vi "ProgramWithConsumerAndProducer.vi"() -> ()   [LabVIEW 2020]
uses:
  #typedef_States.ctl
  <vilib>/picture/picture.llb/imagedata.ctl
  #typedef_Database.ctl
  <vilib>/event_ctls.llb/eventvkey.ctl
  shell32.dll
panel:
  in  "EndOfProgram":bool
  in  "BROWSEINFO 2":T1={"hWndOwner"=0, "pidlRoot"=0, "pszDisplayName"=0, "lpszTitle"=0, "ulFlags"=1, "lpfn"=0, "lParam"=0, "iImage"=0}
  in  "List of images":i32[](listbox)
  in  "Path":string
  out "2D Picture":picture
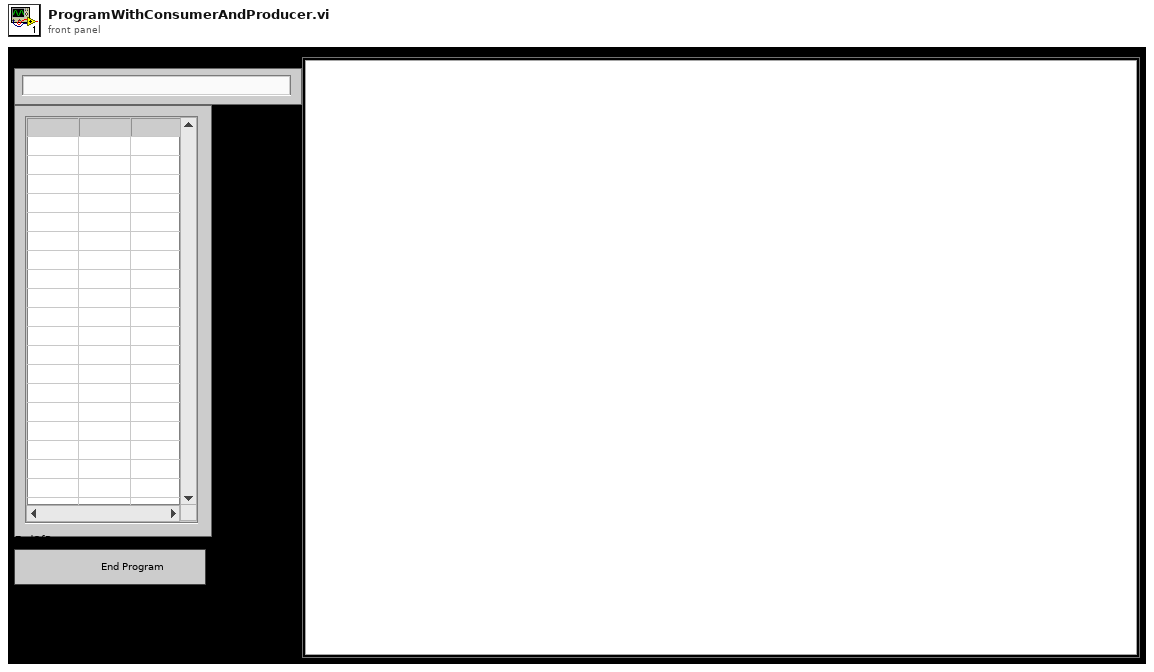
[diagram p1: front panel]
types:
  T1 = cluster{"hWndOwner":i32, "pidlRoot":i32, "pszDisplayName":i32, "lpszTitle":i32, "ulFlags":i32, "lpfn":i32, "lParam":i32, "iImage":i32}
  T2 = typedef "imagedata.ctl" = cluster{"image type":i32, "image depth":i32, "image":u8[], "mask":u8[], "colors":u32[], "Rectangle":cluster{"left":i16, "top":i16, "right":i16, "bottom":i16}}
  T3 = typedef "#typedef_States.ctl" = enum16{"Initialize", "CheckButton", "OpenFromKey", "OpenFromPath", "ImageView", "AreaOfImageResize", "ImageResize", "ChangeImage", "ShowNext", "ShowPrevious", "LoadImagesName", "End"}
  T4 = typedef "#typedef_Database.ctl" = cluster{"Folder Directory":string, "Name of images":string[], "PreviousState":T3, "NumberOfRow":i32, "PanelResizeMeasurement":cluster{"Right":i16, "Left":i16, "Bottom":i16, "Top":i16}, "CurrentImageData":T2, "ImageChangeKey":T5, "IsShiftPressed?":bool}
  T5 = typedef "eventvkey.ctl" = enum16{"ASCII", "Enter", "Return", "Shift", "Ctrl", "Alt", "Cmd", "Opt", "Caps", "NumLock", "Clear", "Break", "Up", "Down", "Left", "Right", "Insert", "Delete", "Home", "End", "PageUp", "PageDown", "Escape", "Help", "Pause", "ScrollLock", "F1", "F2", "F3", "F4", "F5", "F6", "F7", "F8", "F9", "F10", "F11", "F12", "F13", "F14", "F15", "F16", "F17", "F18", "F19", "F20", "F21", "F22", "F23", "F24", "Play", "VolumeUp", "VolumeDown", "Mute", "Two Byte Char"}
  T6 = typedef "LVRectTypeDef.ctl" = cluster{"Left":i16, "Top":i16, "Right":i16, "Bottom":i16}
  T7 = cluster{"Shift":bool, "Ctrl":bool, "Alt":bool, "Cmd":bool, "Opt":bool}
  T8 = typedef "LVBoundsTypeDef.ctl" = cluster{"Width":u32, "Height":u32}
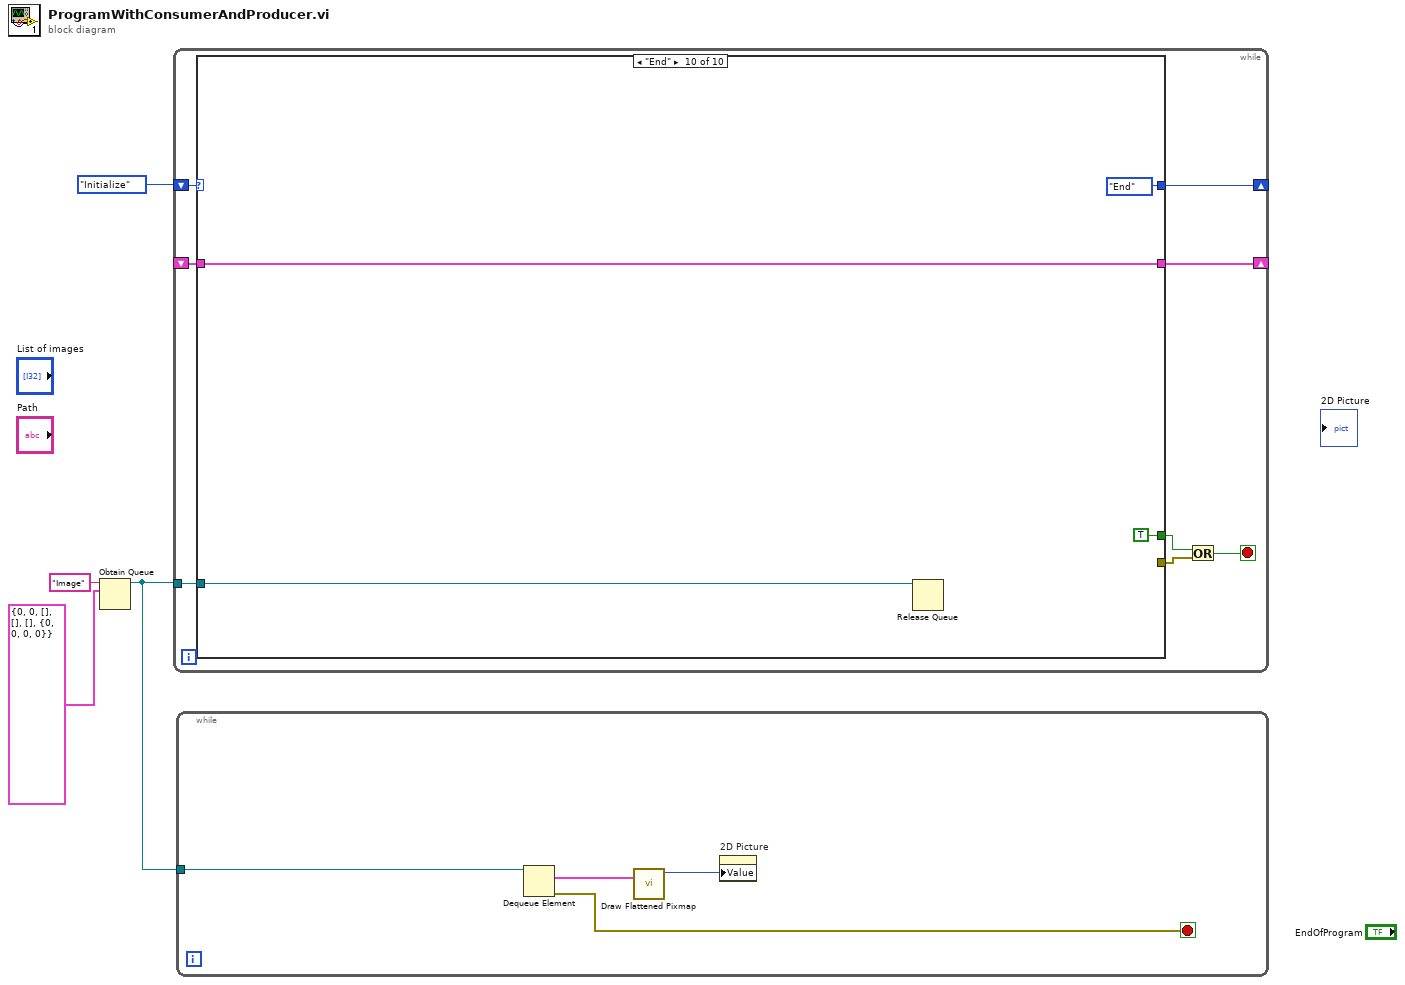
[diagram p0: block diagram]
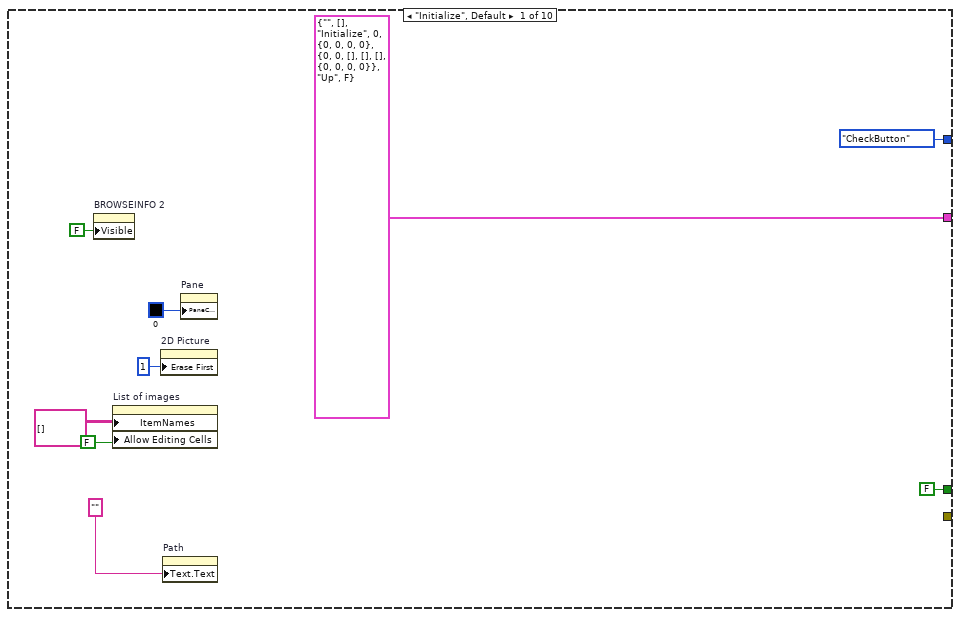
[diagram p2: hidden frame]
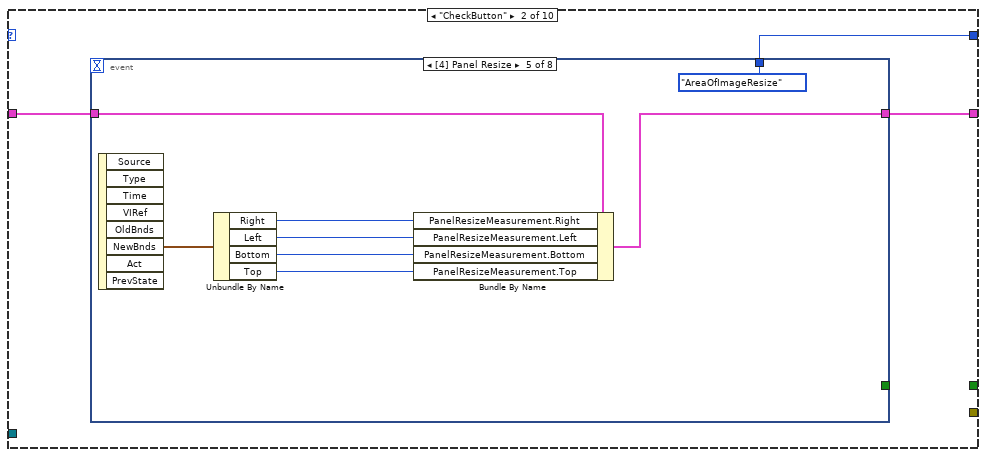
[diagram p3: hidden frame]
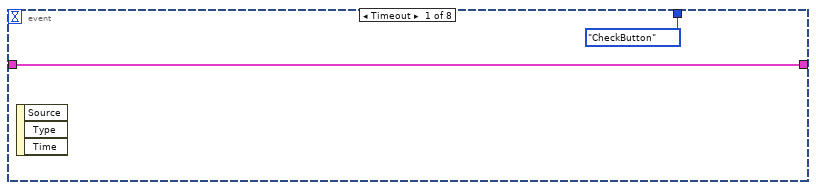
[diagram p4: hidden frame]
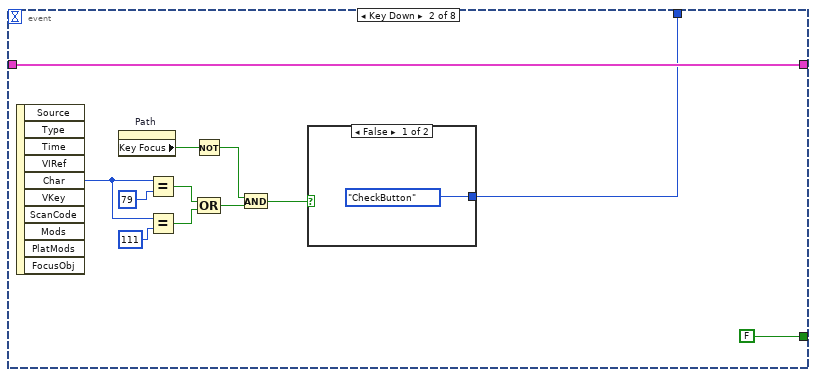
[diagram p5: hidden frame]
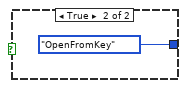
[diagram p6: hidden frame]
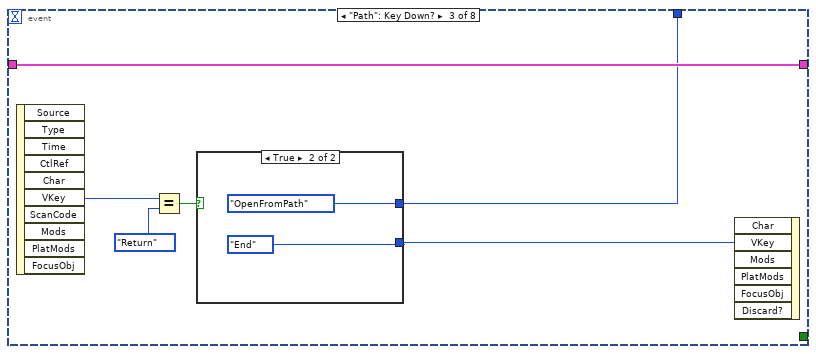
[diagram p7: hidden frame]
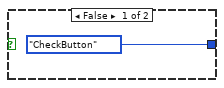
[diagram p8: hidden frame]
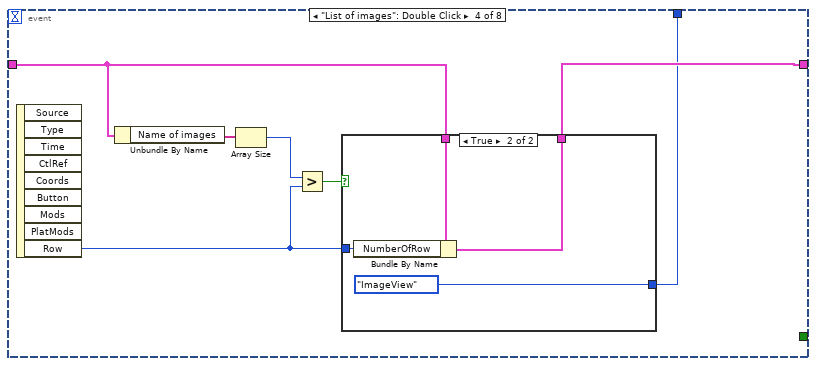
[diagram p9: hidden frame]
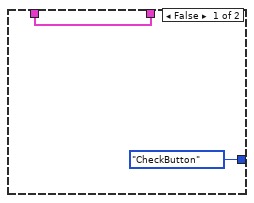
[diagram p10: hidden frame]
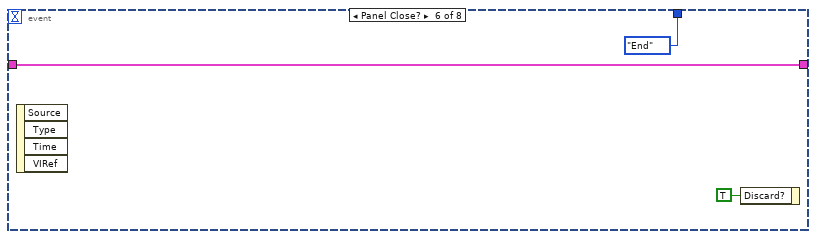
[diagram p11: hidden frame]
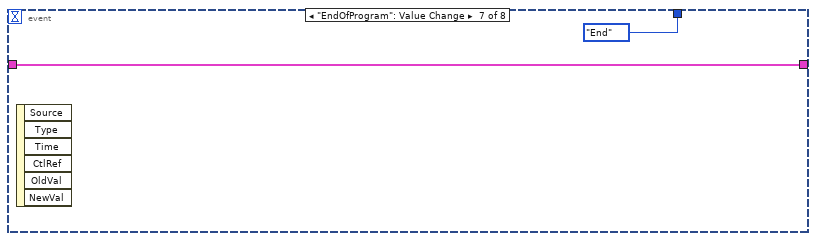
[diagram p12: hidden frame]
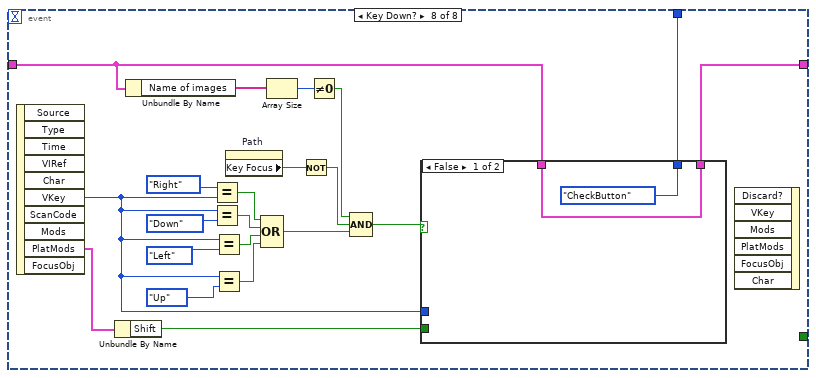
[diagram p13: hidden frame]
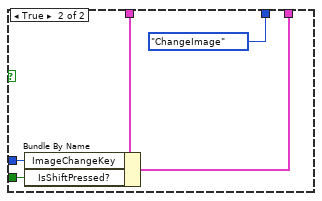
[diagram p14: hidden frame]
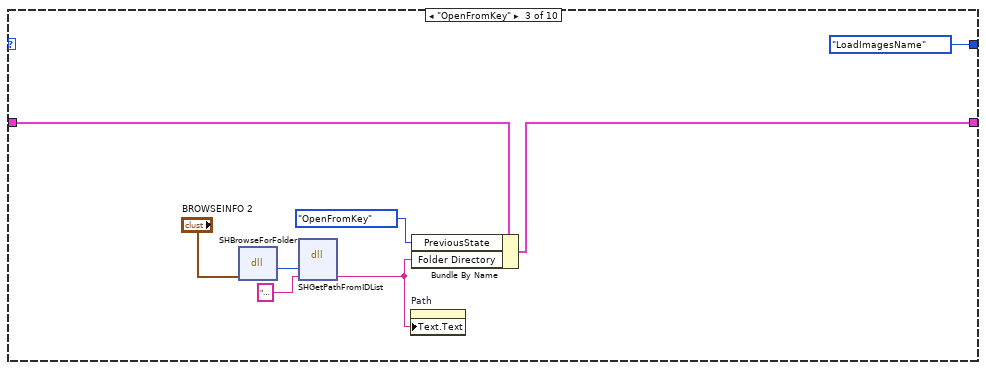
[diagram p15: hidden frame]
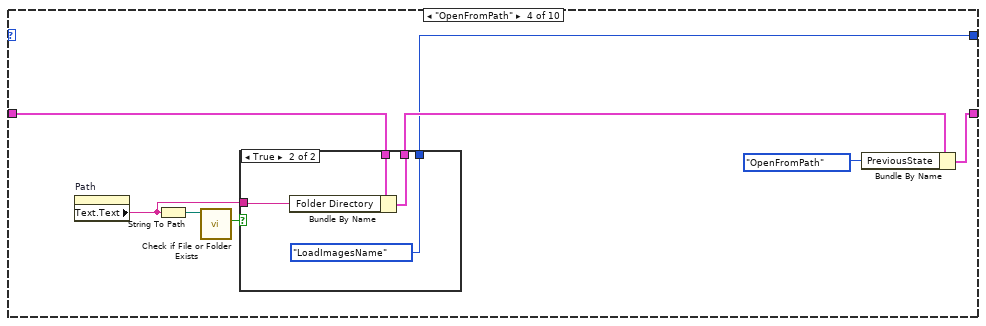
[diagram p16: hidden frame]
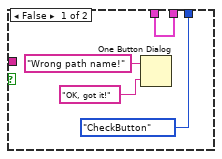
[diagram p17: hidden frame]
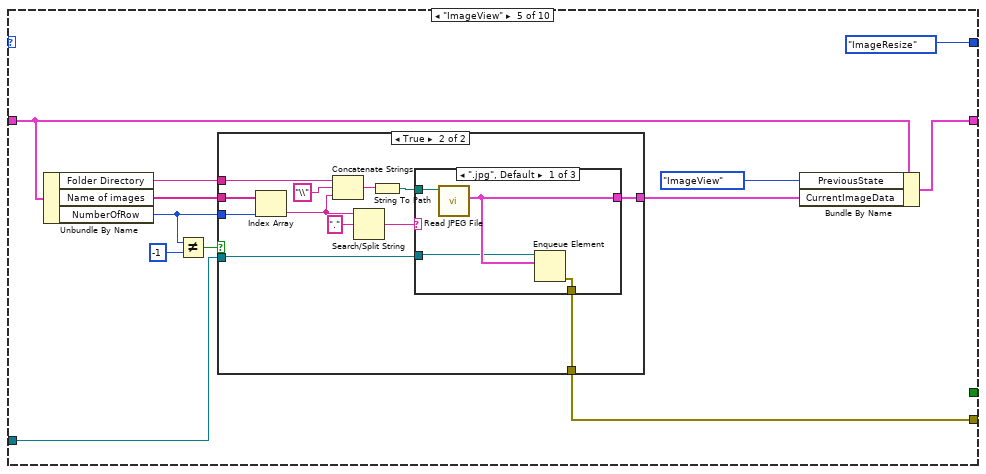
[diagram p18: hidden frame]
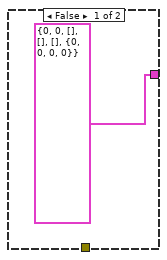
[diagram p19: hidden frame]
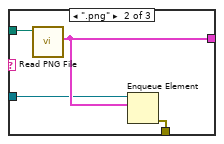
[diagram p20: hidden frame]
diagram:
  n1 = Obtain Queue(name (unnamed)="Image", element data type=T2 {"image type"=0, "image depth"=0, "image"=[], "mask"=[], "colors"=[], "Rectangle"={"left"=0, "top"=0, "right"=0, "bottom"=0}} ("CurrentImageData")) -> (queue out=w1:refnum<queue>)  [unwired: 3 in, 2 out]
  n2 = while {
    shift-right: [w9] -> _
    shift-left: _ -> [w12]
    shift-right: [w10] -> _
    shift-left: #typedef_States."Initialize" ("States") -> [w11]
    tunnel: w1 -> [w8]
    stop <- w5 stop-if-true
    n3 = case shown="\"End\"" w11 {
      tunnel: w12 -> [_ w24 w108 w116 w136 w168 w189 w194 w265 w289]
      tunnel: [T4 {"Folder Directory"="", "Name of images"=[], "PreviousState"=enum."Initialize", "NumberOfRow"=0, "PanelResizeMeasurement"={"Right"=0, "Left"=0, "Bottom"=0, "Top"=0}, "CurrentImageData"={"image type"=0, "image depth"=0, "image"=[], "mask"=[], "colors"=[], "Rectangle"={"left"=0, "top"=0, "right"=0, "bottom"=0}}, "ImageChangeKey"=enum."Up", "IsShiftPressed?"=FALSE} ("Database") w23 w107 w114 w135 w167 w187 w196 w271 w289] -> w9
      tunnel: [#typedef_States."CheckButton" ("States") w22 #typedef_States."LoadImagesName" ("States") w112 #typedef_States."ImageResize" ("States") #typedef_States."ImageResize" ("States") #typedef_States."CheckButton" ("States") #typedef_States."ImageView" ("States") #typedef_States."ImageView" ("States") #typedef_States."End" ("States")] -> w10
      tunnel: w8 -> [_ _ _ _ w129 _ _ _ _ w286]
      tunnel: [FALSE _ _ _ _ _ _ _ _ TRUE] -> w7
      tunnel: [_ _ _ _ w128 _ _ _ _ _] -> w6
      frame "Initialize", Default {
        n4 = property on="BROWSEINFO 2" class="Clust (strict)"("Visible"=FALSE) -> ()  [unwired: 2 in, 2 out]
        n5 = property on="List of images" class="MCListbox (strict)"("ItemNames"=string[][] [] ("Item Names"), "Allow Editing Cells"=FALSE) -> ()  [unwired: 2 in, 2 out]
        n6 = property on="2D Picture" class="Pict"("Erase First"=u8 1) -> ()  [unwired: 2 in, 2 out]
        n7 = property on="Path" class="Str"("Text.Text"="") -> ()  [unwired: 2 in, 2 out]
        n8 = property on="Pane" class="Pane"("PaneColor"=u32 0 ("Pane Color")) -> ()  [unwired: 2 in, 2 out]
      }
      frame "CheckButton" {
        n9 = event shown="[4] Panel Resize" {
          selector: _ -> [_ _ _ _ _ _ _ _]
          dyn-events: _ -> [_ _ _ _ _ _ _ _]
          timeout: _ -> [_ _ _ _ _ _ _ _]
          tunnel: w24 -> [w26 w28 w42 w55 w69 w71 w74 w84]
          tunnel: [w26 w28 w42 w56 w68 w71 w74 w85] -> w23
          tunnel: [_ FALSE _ _ _ _ _ _] -> _
          tunnel: [#typedef_States."CheckButton" ("States") w27 w41 w53 #typedef_States."AreaOfImageResize" ("States") #typedef_States."End" ("States") #typedef_States."End" ("States") w86] -> w22
          event Timeout {
            n10 = event-data() -> ()  [unwired: 1 in, 3 out]
          }
          event Key Down {
            n11 = event-data() -> ("Char"=w38:i16)  [unwired: 1 in, 9 out]
            n12 = property on="Path" class="Str"() -> ("Key Focus"=w32:bool)  [unwired: 2 in, 2 out]
            n13 = Equal?(x=w38, y=i16 79) -> (x = y?=w35:bool)
            n14 = Equal?(x=w38, y=i16 111) -> (x = y?=w34:bool)
            n15 = Not(x=w32) -> (.not. x?=w31:bool)
            n16 = Compound Arithmetic op=OR(w35, w34) -> (w30:bool)
            n17 = And(x=w31, y=w30) -> (x .and. y?=w29:bool)
            n18 = case shown="False" w29 {
              tunnel: [#typedef_States."CheckButton" ("States") #typedef_States."OpenFromKey" ("States")] -> w27
              frame False {
              }
              frame True {
              }
            }
          }
          event "Path": Key Down? {
            n19 = event-data() -> ("VKey"=w45:T5)  [unwired: 1 in, 9 out]
            n20 = Equal?(x=w45, y=eventvkey."Return") -> (x = y?=w46:bool)
            n21 = case shown="True" w46 {
              tunnel: [_ eventvkey."End" ("VKey")] -> w43
              tunnel: [#typedef_States."CheckButton" ("States") #typedef_States."OpenFromPath" ("States")] -> w41
              frame False {
              }
              frame True {
              }
            }
            n22 = event-data("VKey"=w43) -> ()  [unwired: 6 in, 1 out]
          }
          event "List of images": Double Click {
            n23 = event-data() -> ("Row"=w52:i32)  [unwired: 1 in, 8 out]
            n24 = Unbundle By Name(w55) -> ("Name of images"=w54:string[])
            n25 = Array Size(array=w54) -> (size(s)=w50:i32)
            n26 = Greater?(x=w50, y=w52) -> (0:w51:bool)
            n27 = case shown="True" w51 {
              tunnel: w55 -> [w58 w62]
              tunnel: [w58 w61] -> w56
              tunnel: w52 -> [_ w60]
              tunnel: [#typedef_States."CheckButton" ("States") #typedef_States."ImageView" ("States")] -> w53
              frame False {
              }
              frame True {
                n28 = Bundle By Name(cluster=w62, "NumberOfRow"=w60) -> (w61:T4)
              }
            }
          }
          event Panel Resize {
            n29 = event-data() -> ("NewBnds"=w67:T6)  [unwired: 1 in, 7 out]
            n30 = Unbundle By Name(w67) -> ("Right"=w66:i16, "Left"=w65:i16, "Bottom"=w64:i16, "Top"=w63:i16)
            n31 = Bundle By Name(cluster=w69, "PanelResizeMeasurement.Right"=w66, "PanelResizeMeasurement.Left"=w65, "PanelResizeMeasurement.Bottom"=w64, "PanelResizeMeasurement.Top"=w63) -> (w68:T4)
          }
          event Panel Close? {
            n32 = event-data() -> ()  [unwired: 1 in, 4 out]
            n33 = event-data("Discard?"=TRUE) -> ()  [unwired: 1 in, 1 out]
          }
          event "EndOfProgram": Value Change {
            n34 = event-data() -> ()  [unwired: 1 in, 6 out]
          }
          event Key Down? {
            n35 = event-data() -> ("VKey"=w83:T5, "PlatMods"=w77:T7)  [unwired: 1 in, 8 out]
            n36 = Unbundle By Name(w77) -> ("Shift"=w76:bool)
            n37 = Unbundle By Name(w84) -> ("Name of images"=w96:string[])
            n38 = Equal?(x=eventvkey."Right" ("VKey"), y=w83) -> (x = y?=w95:bool)
            n39 = Equal?(x=w83, y=eventvkey."Down" ("VKey")) -> (x = y?=w94:bool)
            n40 = Equal?(x=w83, y=eventvkey."Left" ("VKey")) -> (x = y?=w88:bool)
            n41 = Equal?(x=w83, y=eventvkey."Up" ("VKey")) -> (x = y?=w87:bool)
            n42 = property on="Path" class="Str"() -> ("Key Focus"=w93:bool)  [unwired: 2 in, 2 out]
            n43 = Compound Arithmetic op=OR(w95, w94, w88, w87) -> (w81:bool)
            n44 = Array Size(array=w96) -> (size(s)=w82:i32)
            n45 = Not(x=w93) -> (.not. x?=w80:bool)
            n46 = Not Equal To 0?(x=w82) -> (x != 0?=w79:bool)
            n47 = Compound Arithmetic op=AND(w79, w80, w81) -> (w78:bool)
            n48 = case shown="False" w78 {
              tunnel: [#typedef_States."CheckButton" ("States") #typedef_States."ChangeImage" ("States")] -> w86
              tunnel: w84 -> [w97 w102]
              tunnel: [w97 w101] -> w85
              tunnel: w83 -> [_ w100]
              tunnel: w76 -> [_ w99]
              frame False {
              }
              frame True {
                n49 = Bundle By Name(cluster=w102, "ImageChangeKey"=w100, "IsShiftPressed?"=w99) -> (w101:T4)
              }
            }
            n50 = event-data() -> ()  [unwired: 7 in, 1 out]
          }
        }
      }
      frame "OpenFromKey" {
        n51 = dll-call lib="shell32.dll" fn="SHBrowseForFolder"("BROWSEINFO"="BROWSEINFO 2") -> ("PointerToIDList"=w110:i32)  [unwired: 4 in, 2 out]
        n52 = dll-call lib="shell32.dll" fn="SHGetPathFromIDList"("PointerToIDList"=w110, "PathBuffer"="                                                                                                                                                                                                                                                                    " ("260 char string")) -> ("PathBuffer"=w104:string)  [unwired: 5 in, 2 out]
        n53 = property on="Path" class="Str"("Text.Text"=w104) -> ()  [unwired: 2 in, 2 out]
        n54 = Bundle By Name(cluster=w108, "PreviousState"=#typedef_States."OpenFromKey" ("States"), "Folder Directory"=w104) -> (w107:T4)
      }
      frame "OpenFromPath" {
        n55 = property on="Path" class="Str"() -> ("Text.Text"=w117:string)  [unwired: 2 in, 2 out]
        n56 = String To Path(string=w117) -> (path=w119:path)
        n57 = call <vilib>:"Check if File or Folder Exists.vi"("path"=w119) -> ("file or folder exists?"=w118:bool)  [unwired: 8 in, 2 out]
        n58 = case shown="True" w118 {
          tunnel: w116 -> [w123 w127]
          tunnel: w117 -> [_ w125]
          tunnel: [w123 w126] -> w115
          tunnel: [#typedef_States."CheckButton" ("States") #typedef_States."LoadImagesName" ("States")] -> w112
          frame False {
            n59 = One Button Dialog(message="Wrong path name!", button name ("OK")="OK, got it!") -> ()  [unwired: 1 out]
          }
          frame True {
            n60 = Bundle By Name(cluster=w127, "Folder Directory"=w125) -> (w126:T4)
          }
        }
        n61 = Bundle By Name(cluster=w115, "PreviousState"=#typedef_States."OpenFromPath" ("States")) -> (w114:T4)
      }
      frame "ImageView" {
        n62 = Unbundle By Name(w136) -> ("Folder Directory"=w138:string, "Name of images"=w139:string[], "NumberOfRow"=w131:i32)
        n63 = Not Equal?(x=w131, y=-1) -> (x != y?=w132:bool)
        n64 = case shown="True" w132 {
          tunnel: w139 -> [_ w152]
          tunnel: w138 -> [_ w151]
          tunnel: w131 -> [_ w144]
          tunnel: [T2 {"image type"=0, "image depth"=0, "image"=[], "mask"=[], "colors"=[], "Rectangle"={"left"=0, "top"=0, "right"=0, "bottom"=0}} ("CurrentImageData") w143] -> w133
          tunnel: w129 -> [_ w142]
          tunnel: [_ w141] -> w128
          frame False {
          }
          frame True {
            n65 = Index Array(array=w152, index=w144) -> (element=w149:string)
            n66 = Concatenate Strings(w151, "\\" ("string"), w149) -> (w150:string)
            n67 = Search/Split String(string=w149, search string/char (-)=".") -> (match + rest of string=w148:string)  [unwired: 1 in, 2 out]
            n68 = String To Path(string=w150) -> (path=w147:path)
            n69 = case shown="\".jpg\", Default" w148 {
              tunnel: w147 -> [w156 w160 w164]
              tunnel: [w155 w159 w163] -> w143
              tunnel: w142 -> [w154 w158 w162]
              tunnel: [w153 w157 w161] -> w141
              frame ".jpg", Default {
                n70 = call <vilib>:"Read JPEG File.vi"("path to JPEG file"=w156) -> ("image data"=w155:T2)  [unwired: 8 in, 2 out]
                n71 = Enqueue Element(queue=w154, element=w155) -> (error out=w153:errorcluster)  [unwired: 2 in, 2 out]
              }
              frame ".png" {
                n72 = call <vilib>:"Read PNG File.vi"("path to PNG file"=w160) -> ("image data"=w159:T2)  [unwired: 8 in, 2 out]
                n73 = Enqueue Element(queue=w158, element=w159) -> (error out=w157:errorcluster)  [unwired: 2 in, 2 out]
              }
              frame ".bmp" {
                n74 = call <vilib>:"Read BMP File.vi"("path to BMP file"=w164) -> ("image data"=w163:T2)  [unwired: 8 in, 2 out]
                n75 = Enqueue Element(queue=w162, element=w163) -> (error out=w161:errorcluster)  [unwired: 2 in, 2 out]
              }
            }
          }
        }
        n76 = Bundle By Name(cluster=w136, "PreviousState"=#typedef_States."ImageView" ("States"), "CurrentImageData"=w133) -> (w135:T4)
      }
      frame "AreaOfImageResize" {
        n77 = Unbundle By Name(w168) -> ("PanelResizeMeasurement.Right"=w172:i16, "PanelResizeMeasurement.Left"=w171:i16, "PanelResizeMeasurement.Bottom"=w170:i16, "PanelResizeMeasurement.Top"=w169:i16)
        n78 = Subtract(x=w172, y=w171) -> (x-y=w185:i16)
        n79 = Subtract(x=w170, y=w169) -> (x-y=w184:i16)
        n80 = property on="Path" class="Str"() -> ("Width"=w179:u32)  [unwired: 2 in, 2 out]
        n81 = To Word Integer(number=w179) -> (16bit integer=w176:i16)
        n82 = Subtract(x=w184, y=i16 5) -> (x-y=w181:i16)
        n83 = To Unsigned Long Integer(number=w181) -> (unsigned 32bit integer=w177:u32)
        n84 = Add(x=w176, y=i16 30) -> (x+y=w175:i16)
        n85 = property on="2D Picture" class="Pict"() -> ("Draw Area Size"=w183:T8)  [unwired: 2 in, 2 out]
        n86 = Subtract(x=w185, y=w175) -> (x-y=w182:i16)
        n87 = To Unsigned Long Integer(number=w182) -> (unsigned 32bit integer=w178:u32)
        n88 = Bundle By Name(cluster=w183, "Width"=w178, "Height"=w177) -> (w180:T8)
        n89 = property on="2D Picture" class="Pict"("Draw Area Size"=w180) -> ()  [unwired: 2 in, 2 out]
        n90 = Bundle By Name(cluster=w168, "PreviousState"=#typedef_States."AreaOfImageResize" ("States")) -> (w167:T4)
      }
      frame "ImageResize" {
        n91 = Unbundle By Name(w189) -> ("CurrentImageData"=w190:T2)
        n92 = control-ref of="2D Picture"() -> (w191:refnum<vi>)
        n93 = call "PictureAdjust.vi"("image data"=w190, "Picture in"=w191) -> ("Numeric"=w192:dbl)  [unwired: 9 in]
        n94 = property on="2D Picture" class="Pict"("ZoomFactor"=w192) -> ()  [unwired: 2 in, 2 out]
        n95 = Bundle By Name(cluster=w189, "PreviousState"=#typedef_States."ImageResize" ("States")) -> (w187:T4)
      }
      frame "ChangeImage" {
        n96 = Unbundle By Name(w194) -> ("IsShiftPressed?"=w193:bool)
        n97 = case shown="False" w193 {
          tunnel: w194 -> [w200 w237]
          tunnel: [w199 w236] -> w197
          frame False {
            n98 = Unbundle By Name(w200) -> ("ImageChangeKey"=w205:T5)
            n99 = Equal?(x=eventvkey."Right" ("ImageChangeKey"), y=w205) -> (x = y?=w203:bool)
            n100 = Equal?(x=w205, y=eventvkey."Down" ("ImageChangeKey")) -> (x = y?=w202:bool)
            n101 = Compound Arithmetic op=OR(w203, w202) -> (w201:bool)
            n102 = case shown="True" w201 {
              tunnel: w200 -> [w210 w224]
              tunnel: [w209 w222] -> w199
              frame False {
                n103 = Unbundle By Name(w210) -> ("NumberOfRow"=w208:i32, "Name of images"=w207:string[])
                n104 = Greater?(x=w208, y=0) -> (0:w211:bool)
                n105 = case shown="True" w211 {
                  tunnel: w210 -> [w217 w221]
                  tunnel: [w216 w220] -> w209
                  tunnel: w208 -> [_ w219]
                  tunnel: w207 -> [w214 _]
                  frame False {
                    n106 = Array Size(array=w214) -> (size(s)=w215:i32)
                    n107 = Decrement(x=w215) -> (x-1=w213:i32)
                    n108 = Bundle By Name(cluster=w217, "NumberOfRow"=w213) -> (w216:T4)
                  }
                  frame True {
                    n109 = Decrement(x=w219) -> (x-1=w218:i32)
                    n110 = Bundle By Name(cluster=w221, "NumberOfRow"=w218) -> (w220:T4)
                  }
                }
              }
              frame True {
                n111 = Unbundle By Name(w224) -> ("NumberOfRow"=w223:i32, "Name of images"=w227:string[])
                n112 = Array Size(array=w227) -> (size(s)=w226:i32)
                n113 = Decrement(x=w226) -> (x-1=w225:i32)
                n114 = Less?(x=w223, y=w225) -> (x < y?=w228:bool)
                n115 = case shown="True" w228 {
                  tunnel: w224 -> [w231 w235]
                  tunnel: w223 -> [_ w234]
                  tunnel: [w230 w232] -> w222
                  frame False {
                    n116 = Bundle By Name(cluster=w231, "NumberOfRow"=0) -> (w230:T4)
                  }
                  frame True {
                    n117 = Increment(x=w234) -> (x+1=w233:i32)
                    n118 = Bundle By Name(cluster=w235, "NumberOfRow"=w233) -> (w232:T4)
                  }
                }
              }
            }
          }
          frame True {
            n119 = Unbundle By Name(w237) -> ("ImageChangeKey"=w242:T5)
            n120 = Equal?(x=eventvkey."Right" ("ImageChangeKey"), y=w242) -> (x = y?=w240:bool)
            n121 = Equal?(x=w242, y=eventvkey."Down" ("ImageChangeKey")) -> (x = y?=w239:bool)
            n122 = Compound Arithmetic op=OR(w240, w239) -> (w238:bool)
            n123 = case shown="False" w238 {
              tunnel: w237 -> [w245 w256]
              tunnel: [w244 w255] -> w236
              frame False {
                n124 = Unbundle By Name(w245) -> ("Name of images"=w253:string[], "NumberOfRow"=w247:i32)
                n125 = Array Size(array=w253) -> (size(s)=w252:i32)
                n126 = Subtract(x=w247, y=10) -> (x-y=w246:i32)
                n127 = Decrement(x=w252) -> (x-1=w251:i32)
                n128 = In Range and Coerce(upper limit=w251, x=w246, lower limit=0) -> (coerced(x)=w249:i32)  [unwired: 1 out]
                n129 = Bundle By Name(cluster=w245, "NumberOfRow"=w249) -> (w244:T4)
              }
              frame True {
                n130 = Unbundle By Name(w256) -> ("Name of images"=w263:string[], "NumberOfRow"=w261:i32)
                n131 = Array Size(array=w263) -> (size(s)=w262:i32)
                n132 = Add(x=w261, y=10) -> (x+y=w258:i32)
                n133 = Decrement(x=w262) -> (x-1=w259:i32)
                n134 = In Range and Coerce(upper limit=w259, x=w258, lower limit=0) -> (coerced(x)=w254:i32)  [unwired: 1 out]
                n135 = Bundle By Name(cluster=w256, "NumberOfRow"=w254) -> (w255:T4)
              }
            }
          }
        }
        n136 = Bundle By Name(cluster=w197, "PreviousState"=#typedef_States."ChangeImage" ("States")) -> (w196:T4)
      }
      frame "LoadImagesName" {
        n137 = Unbundle By Name(w265) -> ("Folder Directory"=w274:string)
        n138 = String To Path(string=w274) -> (path=w276:path)
        n139 = for {
          tunnel: w276 -> [w285]
          tunnel: [w283] -> w269 mode=concatenating
          tunnel: string[] ["*.bmp", "*.jpg", "*.png"] -> [w284] mode=indexing
          n140 = List Folder(path=w285, pattern=w284) -> (filenames=w283:string[])  [unwired: 2 in, 3 out]
        }
        n141 = call "ListofImages(name,ext,size).vi"("Folder Directory"=w274, "Name of images"=w269) -> ("List of images (name, ext, size)"=w273:string[][])  [unwired: 9 in]
        n142 = Array Size(array=w269) -> (size(s)=w268:i32)
        n143 = property on="List of images" class="MCListbox (strict)"("ItemNames"=w273, "NumCols"=u32 3 ("Number of Columns")) -> ()  [unwired: 2 in, 2 out]
        n144 = Greater Than 0?(x=w268) -> (x > 0?=w267:bool)
        n145 = case shown="True" w267 {
          tunnel: w265 -> [w278 w282]
          tunnel: [w277 w281] -> w266
          frame False {
            n146 = Bundle By Name(cluster=w278, "NumberOfRow"=-1) -> (w277:T4)
          }
          frame True {
            n147 = Bundle By Name(cluster=w282, "NumberOfRow"=0) -> (w281:T4)
          }
        }
        n148 = Bundle By Name(cluster=w266, "Name of images"=w269, "PreviousState"=#typedef_States."LoadImagesName" ("States")) -> (w271:T4)
      }
      frame "End" {
        n149 = Release Queue(queue=w286) -> ()  [unwired: 2 in, 3 out]
      }
    }
    n150 = Or(x=w7, y=w6) -> (x .or. y?=w5:bool)
  }
  n151 = while {
    tunnel: w1 -> [w292]
    stop <- w290 stop-if-true
    n152 = Dequeue Element(queue=w292) -> (element=w293:T2, error out=w290:errorcluster)  [unwired: 2 in, 2 out]
    n153 = call <vilib>:"Draw Flattened Pixmap.vi"("image data"=w293) -> ("new picture"=w291:picture)  [unwired: 8 in]
    n154 = property on="2D Picture" class="Pict"("Value"=w291) -> ()  [unwired: 2 in, 2 out]
  }
